vi "TestFGVFlag Status.vi"() -> (0 "error out":errorcluster, 2 "Pass":bool)   [LabVIEW 2015]
uses:
  LVClasses/Flags/ColorFlags.ctl
  TypeDef/ActionEnum.ctl
  LVClasses/Flags/Flags.lvclass
panel:
  out "Data Out":string
  in  "State":bool[](array[boolean])=[FALSE, FALSE, FALSE, FALSE]
  out "Flags Read 1":T1={"Flag State"=[1, 3, 5, 7]}
  out "Flags Write":T1={"Flag State"=[1, 3, 5, 7]}
  out "Flags Read 2":T1={"Flag State"=[1, 3, 5, 7]}
  in  "FGV Room":i32=102
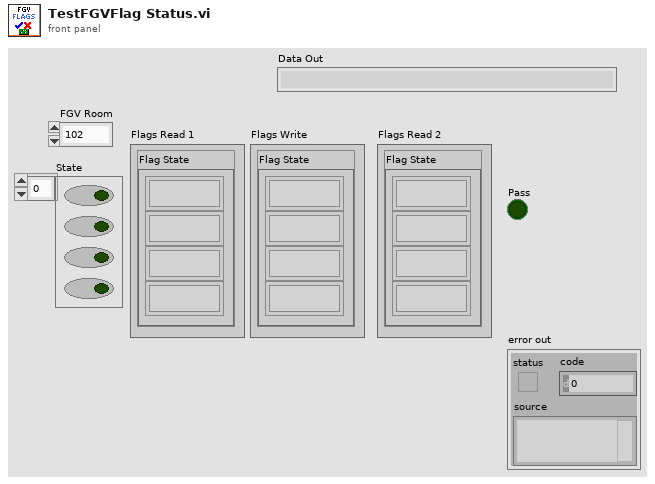
[diagram p1: front panel]
types:
  T1 = typedef "Flags.lvclass/ColorFlags.ctl" = cluster{"Flag State":u8[]}
  T2 = typedef "ActionEnum.ctl" = enum16{"Init", "Add Room", "Remove Room", "Read Room", "Read Flag", "Read Flag State", "Write Flag State", "Read Flag Color", "Write Flag Color", "Read Bed Vacant", "Write Bed Vacant", "Read Personnel", "Add Personnel", "Remove Personnel", "Read Requests", "Add Request", "Remove Request", "Read Beacon ID", "Write Beacon ID", "Write Bed URL", "Read Bed URL"}
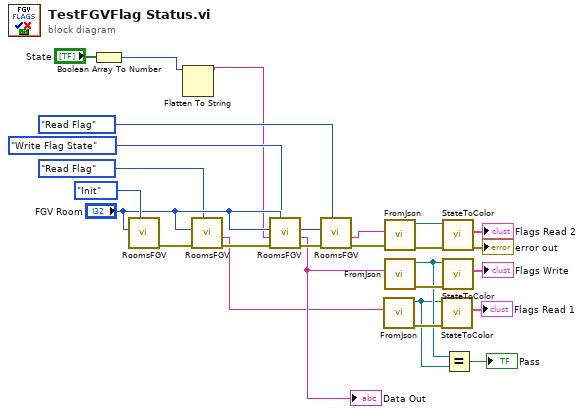
[diagram p0: block diagram]
diagram:
  n1 = Boolean Array To Number(Boolean array="State") -> (number=w1:u32)
  n2 = call "RoomsFGV.vi"("Actions"=ActionEnum."Init", "Room"="FGV Room") -> ("error out"=w24:errorcluster)  [unwired: 8 in, 1 out]
  n3 = Flatten To String(anything=w1) -> (data string=w2:string)  [unwired: 3 in, 2 out]
  n4 = call "RoomsFGV.vi"("Actions"=ActionEnum."Read Flag", "error in (no error)"=w24, "Room"="FGV Room") -> ("error out"=w23:errorcluster, "Data Out"=w9:string)  [unwired: 7 in]
  n5 = call "RoomsFGV.vi"("Actions"=ActionEnum."Write Flag State", "error in (no error)"=w23, "Data In"=w2, "Room"="FGV Room") -> ("error out"=w22:errorcluster, "Data Out"=w10:string)  [unwired: 6 in]
  "Data Out" <- w10
  n6 = call "RoomsFGV.vi"("Actions"=ActionEnum."Read Flag", "error in (no error)"=w22, "Room"="FGV Room") -> ("error out"=w19:errorcluster, "Data Out"=w11:string)  [unwired: 7 in]
  n7 = call "FromJson.vi"("String"=w9) -> ("error out"=w13:errorcluster, "Flags out"=w7:refnum<class "Flags.lvclass">)  [unwired: 9 in]
  n8 = call "FromJson.vi"("error in (no error)"=w19, "String"=w11) -> ("error out"=w17:errorcluster, "Flags out"=w18:refnum<class "Flags.lvclass">)  [unwired: 8 in]
  n9 = call "FromJson.vi"("String"=w10) -> ("error out"=w14:errorcluster, "Flags out"=w8:refnum<class "Flags.lvclass">)  [unwired: 9 in]
  n10 = call "StateToColor.vi"("error in (no error)"=w13, "Flags in"=w7) -> ("RoomNumFlags"=→"Flags Read 1":T1)  [unwired: 7 in, 2 out]
  n11 = call "StateToColor.vi"("error in (no error)"=w17, "Flags in"=w18) -> ("error out"=→"error out":errorcluster, "RoomNumFlags"=→"Flags Read 2":T1)  [unwired: 7 in, 1 out]
  n12 = call "StateToColor.vi"("error in (no error)"=w14, "Flags in"=w8) -> ("RoomNumFlags"=→"Flags Write":T1)  [unwired: 7 in, 2 out]
  n13 = Equal?(x=w8, y=w7) -> (x = y?=→"Pass":bool)
